vi "RSZVB Trace Response Data S-Parameter Group.vi"(8 "error in (no error)":errorcluster {"code" format="%.0x"}, 9 "Data Format (0: Unformatted)":i32(ring) items=["Unformatted", "Formatted", "Unformatted With Trace Mathematics"], 10 "Channel (Trace) (1)":i32=1, 11 "VISA session":refnum<visa-resource-name>) -> (0 "error out":errorcluster {"code" format="%.0x"}, 2 "Trace Data":dbl[](array[numeric]) format="%^.3e", 3 "dup VISA session":refnum<visa-resource-name>)   [LabVIEW 2011]
doc: "This VI reads the current response values of all S-parameters associated to a group of logical ports (S-parameter group). The S-parameter group must be created before using CALCulate<Ch>:PARameter:DEFine:SGRoup.\n\nRemote-control command(s):\nFORMat[:DATA] REAL ,32\nCALCulate<Ch>:DATA:SGRoup? FDATa | SDATa | MDATa"
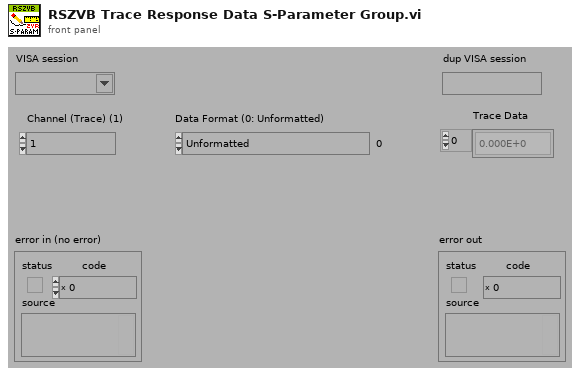
[diagram p1: front panel]
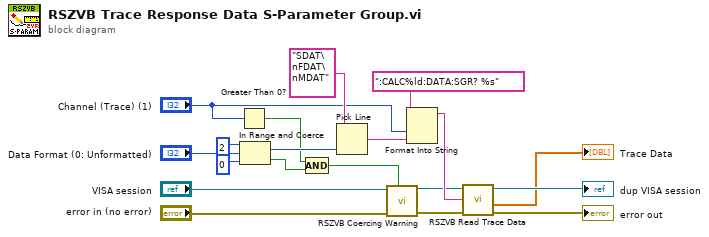
[diagram p0: block diagram]
diagram:
  n1 = Greater Than 0?(x="Channel (Trace) (1)") -> (x > 0?=w10:bool)
  n2 = In Range and Coerce(upper limit=2, x="Data Format (0: Unformatted)", lower limit=0) -> (coerced(x)=w16:i32, In Range?=w9:bool)
  n3 = Compound Arithmetic op=AND(w10, w9) -> (w8:bool)
  n4 = Pick Line(multi-line string="SDAT\nFDAT\nMDAT", line index=w16) -> (output string=w11:string)  [unwired: 1 in]
  n5 = call "RSZVB Coercing Warning.vi"("In Range?"=w8, "error in (no error)"="error in (no error)", "VISA session"="VISA session") -> ("error out"=w4:errorcluster, "dup VISA session"=w5:refnum<visa-resource-name>)  [unwired: 7 in]
  n6 = Format Into String(format string=":CALC%ld:DATA:SGR? %s", "Channel (Trace) (1)", w11) -> (resulting string=w6:string)  [unwired: 2 in, 1 out]
  n7 = call "RSZVB Read Trace Data.vi"("error in (no error)"=w4, "Buffer"=w6, "VISA session"=w5) -> ("error out"=→"error out":errorcluster, "Trace Data"=→"Trace Data":dbl[], "dup VISA session"=→"dup VISA session":refnum<visa-resource-name>)  [unwired: 6 in]
